vi "8to32.vi"(1 "Arrayin":u8[](array[numeric]) format="%x") -> (0 "data32":i32)   [LabVIEW 2018]
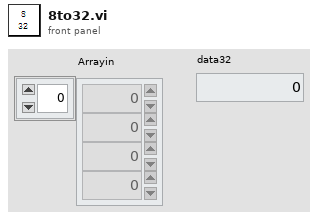
[diagram p1: front panel]
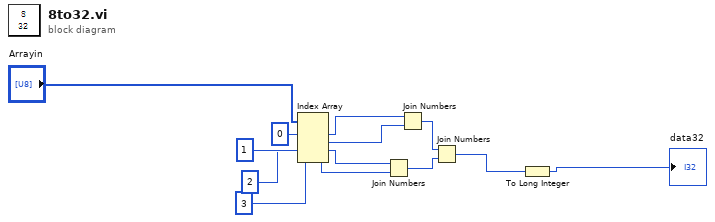
[diagram p0: block diagram]
diagram:
  n1 = Index Array(array="Arrayin", index #1=0 ("索引"), index #2=1 ("索引"), index #3=2 ("索引"), index #4=3 ("索引")) -> (element #1=w3:u8, element #2=w8:u8, element #3=w7:u8, element #4=w6:u8)
  n2 = Join Numbers(hi=w7, lo=w6) -> ((hi.lo)=w4:u16)
  n3 = Join Numbers(hi=w3, lo=w8) -> ((hi.lo)=w5:u16)
  n4 = Join Numbers(hi=w5, lo=w4) -> ((hi.lo)=w2:u32)
  n5 = To Long Integer(number=w2) -> (32bit integer=→"data32":i32)
